vi "Make Terminals Required.vi"(8 "error in (no error)":errorcluster, 10 "Required Terms":i32[](array[numeric]), 11 "VI Reference In":refnum<vi>) -> (0 "error out":errorcluster, 3 "VI Reference Out":refnum<vi>)   [LabVIEW 2021]
panel:
  # "This VI takes a reference to the scripted VI and marks terminals in the Required Terms input as required on the \nscripted VI connector pane"
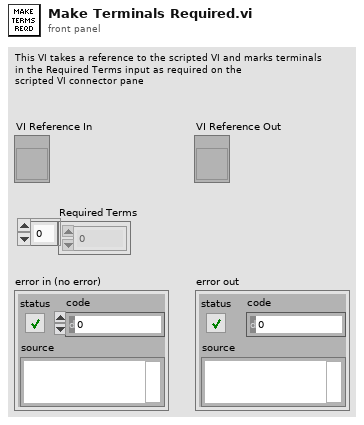
[diagram p1: front panel]
types:
  T1 = enum16{"Invalid Wire Rule", "Required", "Recommended", "Optional", "Dynamic Dispatch"}[]
  T2 = enum16{"Invalid Wire Rule", "Required", "Recommended", "Optional", "Dynamic Dispatch"}
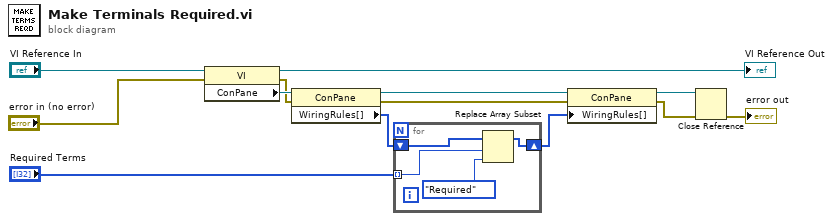
[diagram p0: block diagram]
diagram:
  n1 = property class="VI"(reference="VI Reference In", error in="error in (no error)") -> (reference out=→"VI Reference Out":refnum<vi>, error out=w4:errorcluster, "ConPane"=w8:refnum<vi>)
  n2 = property class="ConPane"(reference=w8, error in=w4) -> (reference out=w12:refnum<vi>, error out=w5:errorcluster, "WiringRules[]"=w9:T1)
  n3 = for {
    tunnel: "Required Terms" -> [w16] mode=indexing
    shift-right: [w14] -> w11
    shift-left: w9 -> [w17]
    n4 = Replace Array Subset(array=w17, new element=T2."Required" ("new element/subarray"), index=w16) -> (w14:T1)
  }
  n5 = property class="ConPane"(reference=w12, error in=w5, "WiringRules[]"=w11) -> (reference out=w7:refnum<vi>, error out=w6:errorcluster)
  n6 = Close Reference(reference=w7, error in (no error)=w6) -> (error out=→"error out":errorcluster)
